vi "Configure IO Trigin Source.vi"(8 "error in (no error)":errorcluster, 10 "Type(0:Meter)":u16(ring) items=["Meter", "Dlog", "List"], 11 "VISA resource name":refnum<visa-resource-name>) -> (0 "error out":errorcluster, 3 "VISA resource name out":refnum<visa-resource-name>)   [LabVIEW 2020, in "IT6000C.lvlib"]
doc: "This command sets the type of the number IO4 trig.\n\n<b>Type</b>\n0:METEr\n1:DLOG\n2:LIST"
uses:
  IT6000C.lvlib
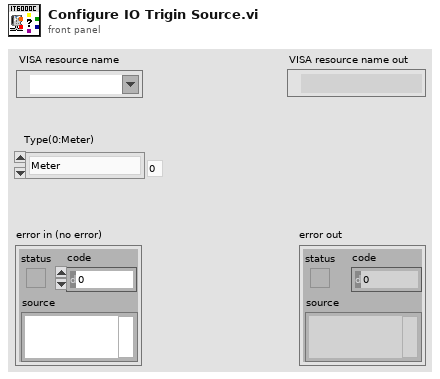
[diagram p1: front panel]
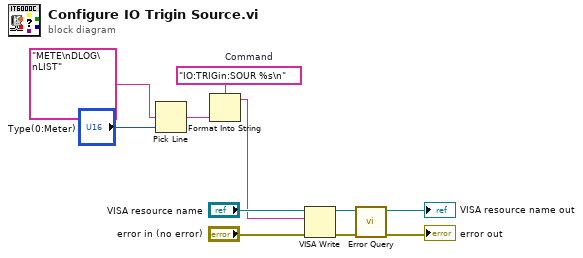
[diagram p0: block diagram]
diagram:
  w5 = "IO:TRIGin:SOUR %s\n"  # Command
  n1 = Pick Line(multi-line string="METE\nDLOG\nLIST", line index="Type(0:Meter)") -> (output string=w1:string)  [unwired: 1 in]
  n2 = Format Into String(format string=w5, w1) -> (resulting string=w4:string)  [unwired: 2 in, 1 out]
  n3 = VISA Write(VISA resource name="VISA resource name", write buffer=w4, error in (no error)="error in (no error)") -> (VISA resource name out=w8:refnum<visa-resource-name>, error out=w9:errorcluster)  [unwired: 1 out]
  n4 = call "Error Query.vi"("error in (no error)"=w9, "VISA resource name"=w8) -> ("error out"=→"error out":errorcluster, "VISA resource name out"=→"VISA resource name out":refnum<visa-resource-name>)  [unwired: 6 in, 2 out]
